vi "Sector to graph.vi"(10 "Sector":dbl=0.1) -> (2 "XY Graph":cluster{dbl[], dbl[]}(graph))   [LabVIEW 2009]
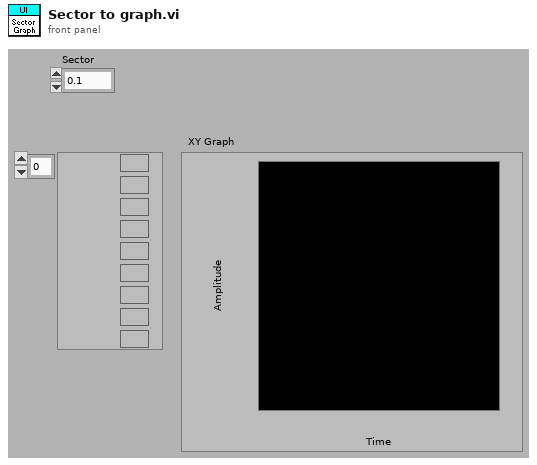
[diagram p1: front panel]
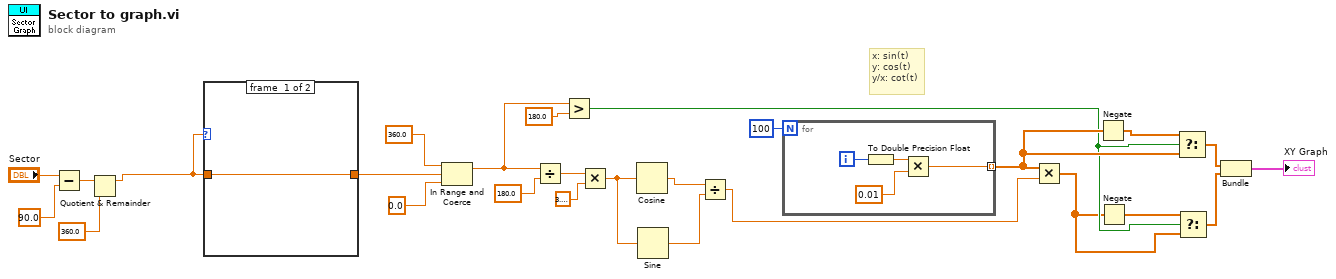
[diagram p0: block diagram]
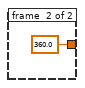
[diagram p2: hidden frame]
diagram:
  # "x: sin(t)\ny: cos(t)\ny/x: cot(t)"
  n1 = Subtract(x="Sector", y=90.0) -> (x-y=w3:dbl)
  n2 = Quotient & Remainder(x=w3, y=360.0) -> (x-y*floor(x/y)=w1:dbl)  [unwired: 1 out]
  n3 = case shown="Default" w1 {
    tunnel: [w27 360.0 ("Bearing")] -> w18
    tunnel: w1 -> [w27 _]
    frame #0 {
    }
    frame #1 {
    }
  }
  n4 = In Range and Coerce(upper limit=360.0, x=w18, lower limit=0.0) -> (coerced(x)=w15:dbl)  [unwired: 1 out]
  n5 = Divide(x=w15, y=180.0) -> (x/y=w24:dbl)
  n6 = Greater?(x=w15, y=180.0) -> (0:w9:bool)
  n7 = Multiply(x=w24, y=3.141592653589793) -> (x*y=w22:dbl)
  n8 = Cosine(x=w22) -> (cos(x)=w20:dbl)
  n9 = Sine(x=w22) -> (sin(x)=w19:dbl)
  n10 = Divide(x=w20, y=w19) -> (x/y=w21:dbl)
  n11 = for {
    N: 100 -> [_]
    tunnel: [w29] -> w12 mode=indexing
    i -> [w32]
    n12 = To Double Precision Float(number=w32) -> (double precision float=w31:dbl)
    n13 = Multiply(x=w31, y=0.01) -> (x*y=w29:dbl)
  }
  n14 = Multiply(x=w12, y=w21) -> (x*y=w8:dbl[])
  n15 = Negate(x=w12) -> (-x=w13:dbl[])
  n16 = Negate(x=w8) -> (-x=w10:dbl[])
  n17 = Select(t=w13, s=w9, f=w12) -> (s? t:f=w11:dbl[])
  n18 = Select(t=w10, s=w9, f=w8) -> (s? t:f=w7:dbl[])
  n19 = Bundle(w11, w7) -> (→"XY Graph":cluster{dbl[], dbl[]})  [unwired: 1 in]
